vi "Monitor for Stop.vi"(8 "error in (no error)":errorcluster, 10 "service stop events":refnum<user-event>[](array[refnum]), 11 "Event Registration Refnum in":refnum<event-registration>) -> (0 "error out":errorcluster, 3 "Event Registration Refnum out":refnum<event-registration>)   [LabVIEW 2025, in "Automotive-Vision-OOBService_server.lvlib"]
uses:
  Automotive-Vision-OOBService_server.lvlib
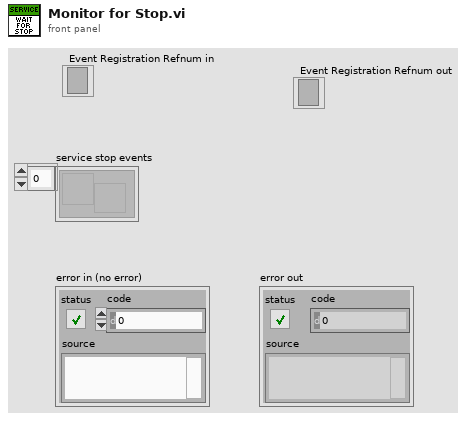
[diagram p1: front panel]
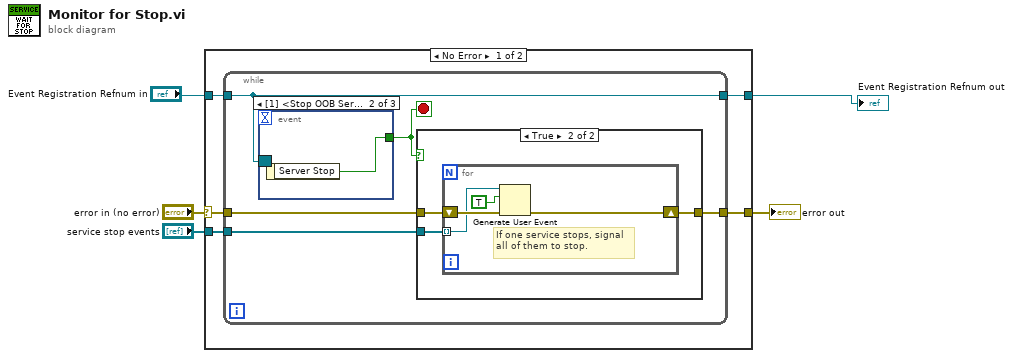
[diagram p0: block diagram]
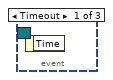
[diagram p2: hidden frame]
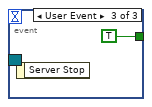
[diagram p3: hidden frame]
diagram:
  n1 = case shown="No Error" "error in (no error)" {
    selector: "error in (no error)" -> [w8 w27]
    tunnel: "Event Registration Refnum in" -> [w10 w26]
    tunnel: "service stop events" -> [w9 _]
    tunnel: [w6 w27] -> w5
    tunnel: [w7 w26] -> w1
    frame No Error {
      n2 = while {
        tunnel: w10 -> [w12]
        tunnel: [w12] -> w7
        tunnel: [w13] -> w6
        tunnel: w9 -> [w14]
        tunnel: w8 -> [w15]
        stop <- w11 stop-if-true
        n3 = event shown="[1] <Stop OOB Server UE>: User Event" {
          selector: w12 -> [_ _ _]
          dyn-events: _ -> [_ _ _]
          timeout: _ -> [_ _ _]
          tunnel: [_ w16 TRUE] -> w11
          event Timeout {
            n4 = event-data() -> ()  [unwired: 1 in, 1 out]
          }
          event User Event {
            n5 = event-data() -> ("Server Stop"=w16:bool)  [unwired: 1 in]
          }
          event User Event {
            n6 = event-data() -> ()  [unwired: 1 in, 1 out]
          }
        }
        n7 = case shown="True" w11 {
          tunnel: w15 -> [w18 w21]
          tunnel: w14 -> [_ w20]
          tunnel: [w18 w19] -> w13
          frame False {
          }
          frame True {
            n8 = for {
              shift-right: [w24] -> w19
              shift-left: w21 -> [w23]
              tunnel: w20 -> [w22] mode=indexing
              # "If one service stops, signal\nall of them to stop."
              n9 = Generate User Event(user event=w22, event data cluster=TRUE ("event data"), error in=w23) -> (error out=w24:errorcluster)  [unwired: 1 in, 1 out]
            }
          }
        }
      }
    }
    frame Error {
    }
  }
  "error out" <- w5
  "Event Registration Refnum out" <- w1
